vi "Test Parser.vi"() -> ()   [LabVIEW 2019, in "PGC2D.lvlib"]
uses:
  PGC2D.lvlib
panel:
  out "error out":errorcluster
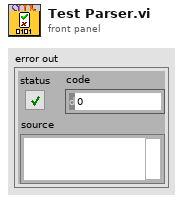
[diagram p1: front panel]
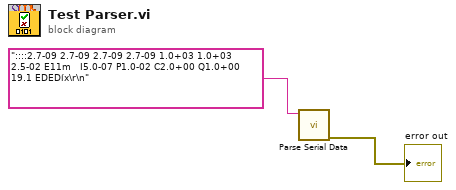
[diagram p0: block diagram]
diagram:
  n1 = call "Parse Serial Data.vi"("Buffer in"="::::2.7-09 2.7-09 2.7-09 2.7-09 1.0+03 1.0+03 2.5-02 E11m   I5.0-07 P1.0-02 C2.0+00 Q1.0+00 19.1 EDEDíx\r\n") -> ("error out"=→"error out":errorcluster)  [unwired: 8 in, 2 out]
